vi "InitStack.vi"(9 "Action Stack":refnum<class "Action.lvclass">[](array[class])) -> (1 "Stack":refnum<class "Stack.lvclass">)   [LabVIEW 2024, in "ActionStack.lvlib" / "Stack.lvclass"]
uses:
  Stack.lvclass
  Action/Action.lvclass
  Stack.lvclass/Stack.ctl
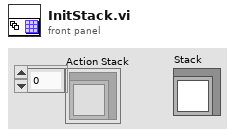
[diagram p1: front panel]
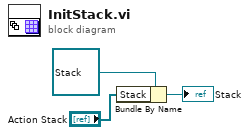
[diagram p0: block diagram]
diagram:
  n1 = Bundle By Name(cluster=refnum<class "Stack.lvclass"> refnum ("Stack.lvclass"), "Stack"="Action Stack") -> (→"Stack":refnum<class "Stack.lvclass">)
